vi "PDF_Interface_PDF Protokoll EPA1065_520 Pre Test.vi"(8 "error in (no error)":errorcluster caption="Fehler (Eingang, kein Fehler)", 10 "ResultPictures":T1, 11 "Save PDF File Path":path) -> (0 "error out":errorcluster caption="Fehler (Ausgang)")   [LabVIEW 2020, in "EPA 1065.lvlib" / "Pre-test verification 1065-520.lvlib"]
uses:
  Pre-test verification 1065-520.lvlib
  T90 1065-308/Ergebnis.ctl
  PDF_Interface/PDF Interface Helper/PDFResultPictures.ctl
  Sprachverwaltung/FGV Aktion Tabelle zerlegen.ctl
  Seiten/FT-IR/FGV FT-IR Aktionen.ctl
  Seiten/System Einstellungen V2/Aktioen FGV System Konstanten.ctl
  Aktion FGV Pre Test Daten.ctl
  PDF_Interface/PDF Protokoll Standard Kopf Optionen.ctl
  <vilib>/Simplicity AI/SAI_PDF_API/Classes/Context/Controls/SAI_PDF_PDF Details.ctl
  PDF_Interface/PDF Interface Helper/PDFContentType.ctl
  PDF_Interface/PDF Interface Helper/PDFTableContentType.ctl
  PDF_Interface/PDF Interface Helper/PDFResults.ctl
  PDF_Interface/PDF Interface Helper/PDFCommentPosition.ctl
  PDF_Interface/PDF Interface Helper/PDFPageBreak.ctl
  PDF_Interface/PDF Interface Helper/PDFTablePictures.ctl
  PDF_Interface/PDF Interface Helper/PDFBemerkung.ctl
  <vilib>/Simplicity AI/SAI_PDF_API/Classes/Context/Controls/SAI_PDF_Text Align.ctl
  <vilib>/Simplicity AI/SAI_PDF_API/Classes/Context/Controls/SAI_PDF_Font.ctl
  <vilib>/Simplicity AI/SAI_PDF_API/Classes/Context/Controls/SAI_PDF_Font Encoding.ctl
  Allgemein/allgemeine Sub-VIs.lvlib
  Seiten/FT-IR/FT-IR.lvlib
  Seiten/System Einstellungen V2/System Einstellungen V2.lvlib
  Sprachverwaltung/Sprachverwaltung.lvlib
  PDF_Interface/PDF Interface.lvlib
  PDF_Interface/PDF Interface Helper/PDF Interface Helper.lvlib
  <vilib>/Simplicity AI/SAI_PDF_API/Classes/Context/Context.lvclass
  Linearisierung V2/Protokoll/Protokoll.lvlib
  T90 1065-308/T90 Test 1065-308.lvlib
panel:
  out "Einheit Genauigkeit 2":string
  out "Ergebnis":T2 caption="Ergebnis 1"
  out "Ergebnis THC":string
  out "Grenze":string caption="Grenzwert:"
  out "Einheit Genauigkeit":string
  out "Versa Serial number:":string caption="Seriennummer:"
  out "Anlage:":string
  out "Methode (Recipe):":string
  out "Date & Time:":string caption="Datum & Uhrzeit:"
  out "Ergebnis:":string
  out "Flow weighted mean:":string caption="Durchflussgew. Mittelwert:"
  out "Bearbeiter:":string
  out "Serial number:":string caption="Seriennummer:"
  out "Messgerät:":string
  # "Pre Test EPA § 1065.520"
  # "Grenzen"
  # "Ergebnis"
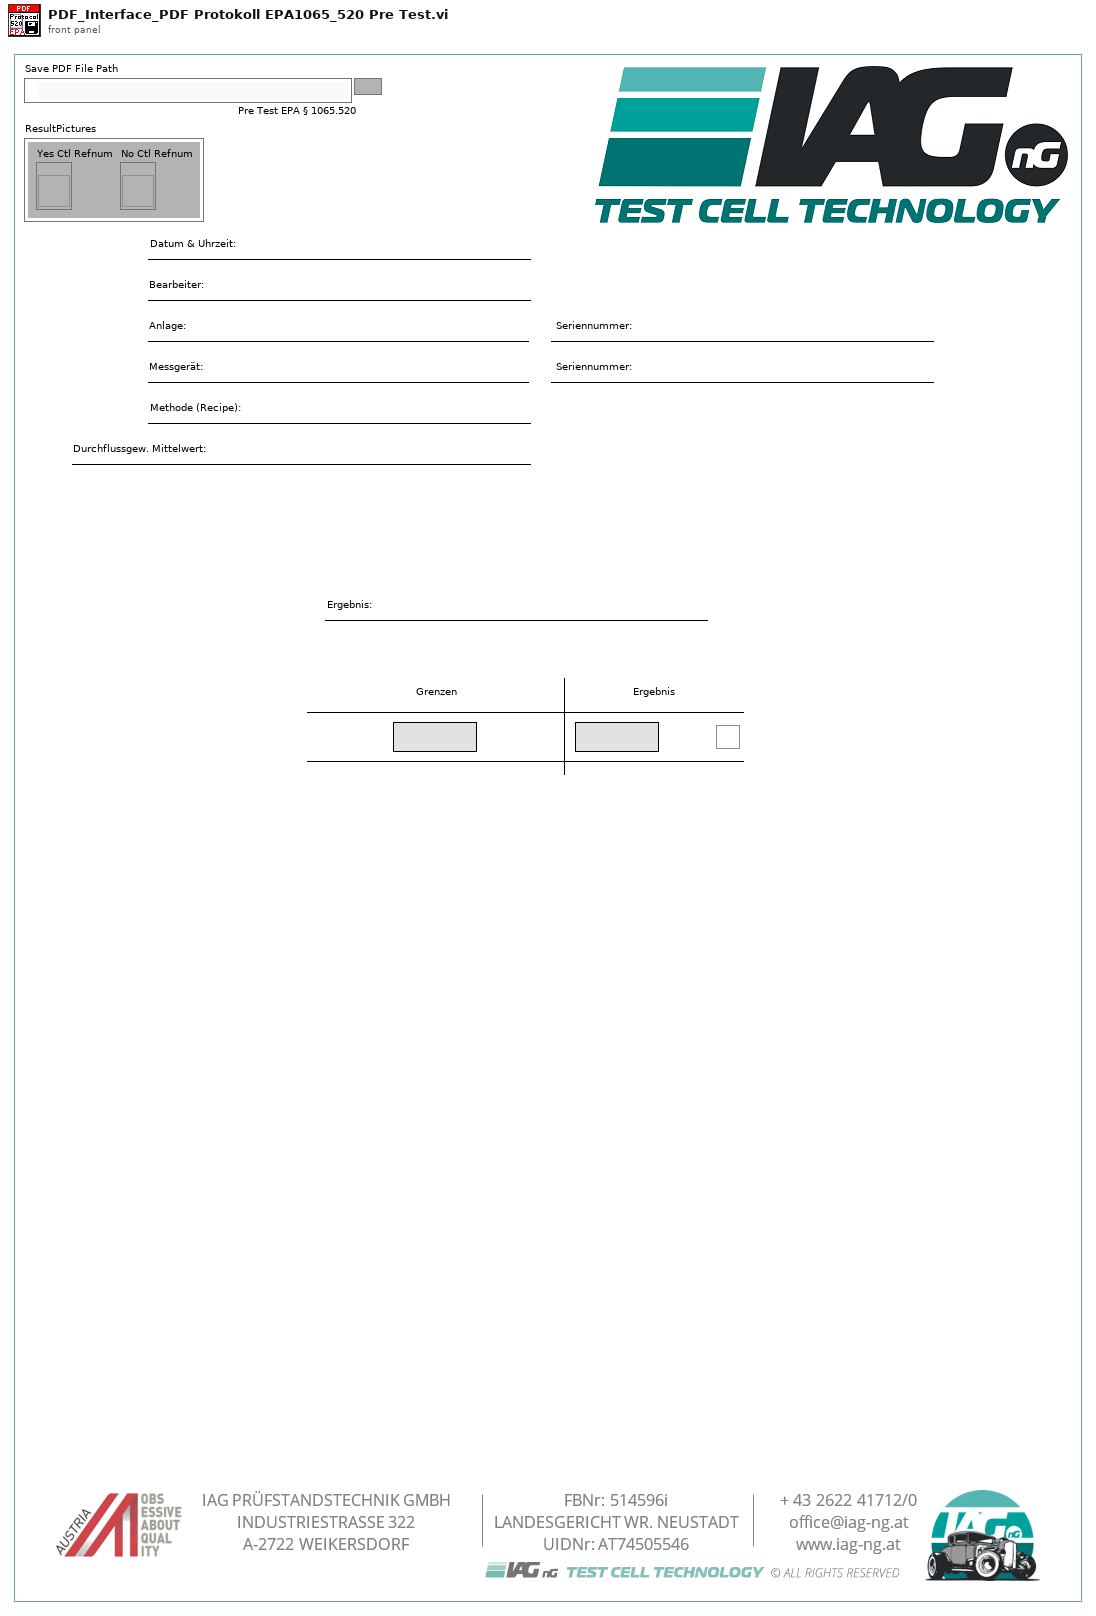
[diagram p1: front panel]
types:
  T1 = typedef "PDF Interface.lvlib/PDF Interface Helper.lvlib/PDFResultPictures.ctl" = cluster{"Yes Ctl Refnum":refnum<vi>, "No Ctl Refnum":refnum<vi>}
  T2 = typedef "EPA 1065.lvlib/T90 Test 1065-308.lvlib/Ergebnis.ctl" = bool
  T3 = typedef "Sprachverwaltung.lvlib/FGV Aktion Tabelle zerlegen.ctl" = enum16{"laden", "vereinzeln", "speichern"}
  T4 = typedef "PDF Interface.lvlib/PDF Protokoll Standard Kopf Optionen.ctl" = cluster{"Analysator":bool, "FT-IR Rezept":bool, "Gasteiler":bool, "Gas Komponente":bool, "Gas Flasche":bool, "LIN Protokoll":bool, "Operator":bool}
  T5 = typedef "EPA 1065.lvlib/Pre-test verification 1065-520.lvlib/Aktion FGV Pre Test Daten.ctl" = enum16{"lesen", "Konfig Daten", "PDF einstellen", "laden", "speichern", "Werte schreiben", "Auswerten"}
  T6 = typedef "System Einstellungen V2.lvlib/Aktioen FGV System Konstanten.ctl" = enum16{"lesen", "laden", "speichern", "Sprache"}
  T7 = typedef "FT-IR.lvlib/FGV FT-IR Aktionen.ctl" = enum16{"lesen", "NOG setzen", "NOS setzen", "Initialisieren", "speichern", "ALLES setzen", "FT-IR Spektrum loggen", "Komm Stoppen", "Spektrum LogKonfig"}
  T8 = typedef "PDF Interface.lvlib/PDF Interface Helper.lvlib/PDFResults.ctl" = cluster{"Results":cluster{"Result Text":string, "Result":bool}[], "ResultPictures":T1, "use Pictures":bool, "Image Scale (%)":sgl, "Autoscale? (T)":bool, "Horizontal Align":i32, "Position":i32}
  T9 = typedef "PDF Interface.lvlib/PDF Interface Helper.lvlib/PDFTableContentType.ctl" = cluster{"TableHeader":string[], "Table":string[][], "Relative Column Widths (%)":sgl[], "Results":T8, "PositionBemerkung":T10, "PageBreak":T11, "TablePictures":T12, "Horizontal Align":i32}
  T10 = typedef "PDF Interface.lvlib/PDF Interface Helper.lvlib/PDFCommentPosition.ctl" = enum16{"before", "after"}
  T11 = typedef "PDF Interface.lvlib/PDF Interface Helper.lvlib/PDFPageBreak.ctl" = enum16{"none", "before", "after", "after comment"}
  T12 = typedef "PDF Interface.lvlib/PDF Interface Helper.lvlib/PDFTablePictures.ctl" = cluster{"Ctl Refnum In":refnum<vi>[], "RowOrColumn":enum16{"Row", "Column"}, "IndexToInsert":u16, "Image Scale (%)":sgl[], "Autoscale? (T)":bool[], "Horizontal Align":i32}
  T13 = typedef "PDF Interface.lvlib/PDF Interface Helper.lvlib/PDFBemerkung.ctl" = cluster{"Bemerkung Text":string, "Align (Left)":T14, "Add Line Feeds (F:No)":bool, "Font":T15}
  T14 = typedef "SAI_PDF_Toolkit.lvlib/Context.lvclass/SAI_PDF_Text Align.ctl" = i32
  T15 = typedef "SAI_PDF_Toolkit.lvlib/Context.lvclass/SAI_PDF_Font.ctl" = cluster{"Font":string, "Size":i32, "Colour":u32, "Bold":bool, "Italic":bool, "Underline":bool, "Strikethrough":bool, "Font Encoding":T16}
  T16 = typedef "SAI_PDF_Toolkit.lvlib/Context.lvclass/SAI_PDF_Font Encoding.ctl" = enum16{"Cp1252, WinANSI", "IdentityH", "IdentityV", "Cp1250", "Cp1257", "MacRoman"}
  T17 = typedef "PDF Interface.lvlib/PDF Interface Helper.lvlib/PDFContentType.ctl" = cluster{"Titel":string, "Header Table":string[][], "Table Array":T9[], "Bemerkungen":T13[]}
  T18 = typedef "SAI_PDF_Toolkit.lvlib/Context.lvclass/SAI_PDF_PDF Details.ctl" = cluster{"Title":string, "Subject":string, "Keywords":string, "Author":string, "Creator":string}
  T19 = cluster{"Header Footer Text Cluster":cluster{"Header Text":string, "Footer Text":string, "Time":string, "Page Number":string}, "PDF Details":T18}
  T20 = typedef "EPA 1065.lvlib/Pre-test verification 1065-520.lvlib/Pre Konfig Daten.ctl" = cluster{"Bearbeiter:":string, "Messgerät:":string, "Seriennummer:":string, "Modus":T21, "Pfad:":path, "Textname:":string, "N2 Aufschaltzeit:":dbl, "Flow weighted mean:":dbl}
  T21 = typedef "EPA 1065.lvlib/Pre-test verification 1065-520.lvlib/Modus Pre Test.ctl" = u16
  T22 = cluster{"Modell":string, "ProjektNummer":string, "Software Version":string, "Seriennummer":string}
  T23 = cluster{"Header Size":i32, "Column Ratio left":sgl[]}
  T24 = typedef "String - Ausgabefeld.ctl" = string
  T25 = typedef "EPA 1065.lvlib/Pre-test verification 1065-520.lvlib/Pre Werte.ctl" = cluster{"THC Wert":dbl, "Berechnetes Limit":dbl, "Bestanden":bool}
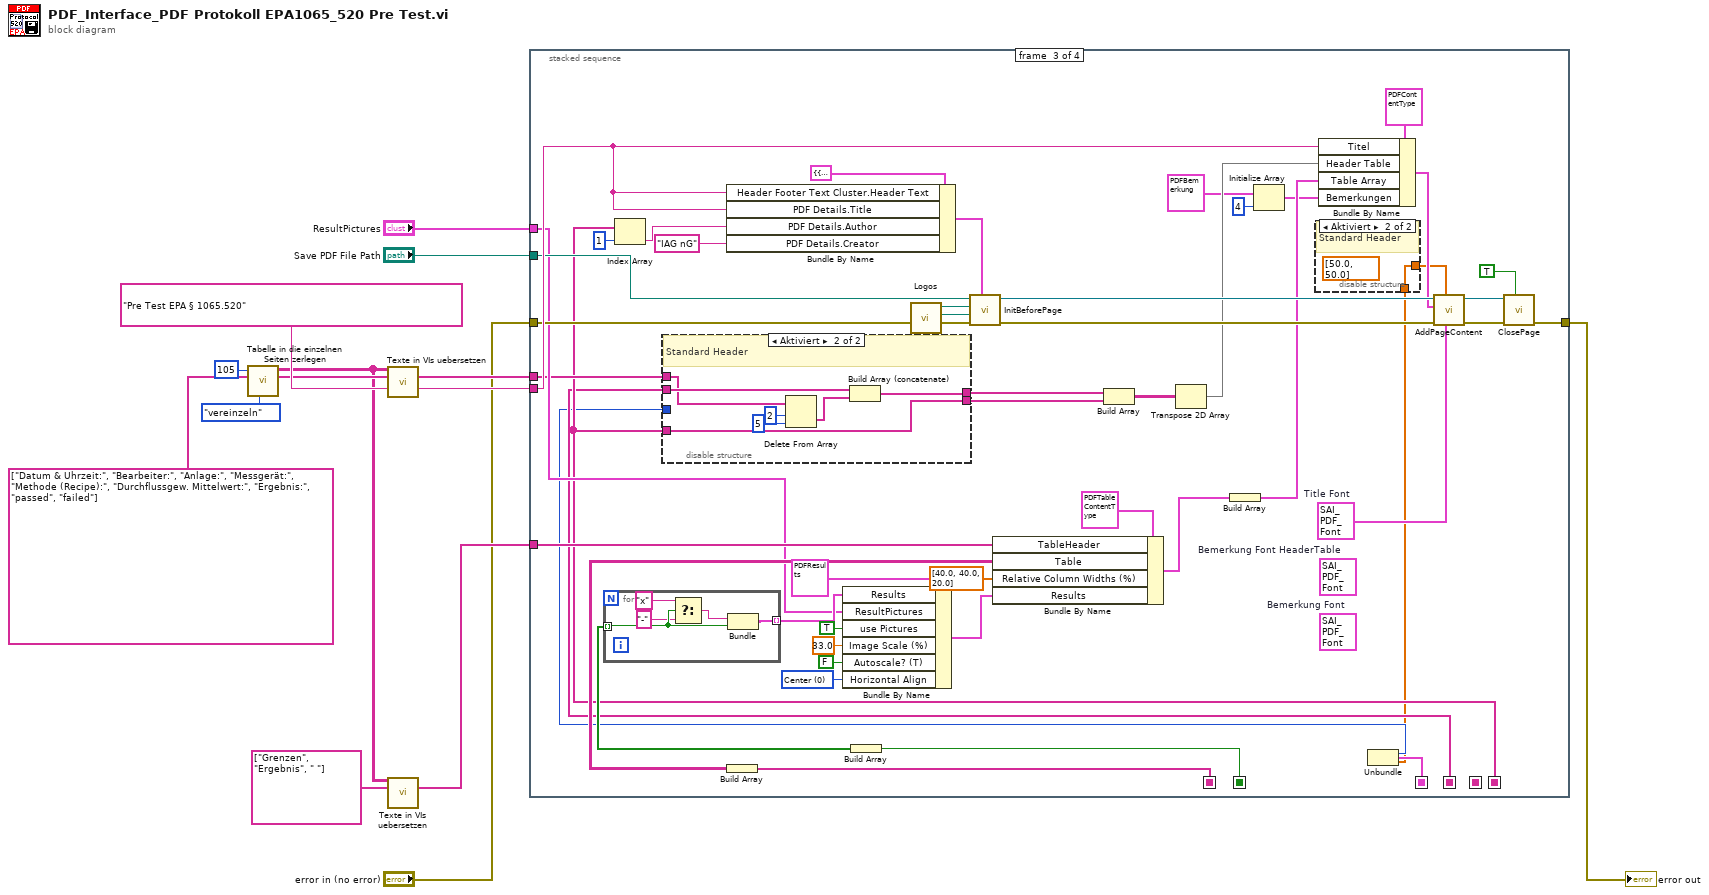
[diagram p0: block diagram]
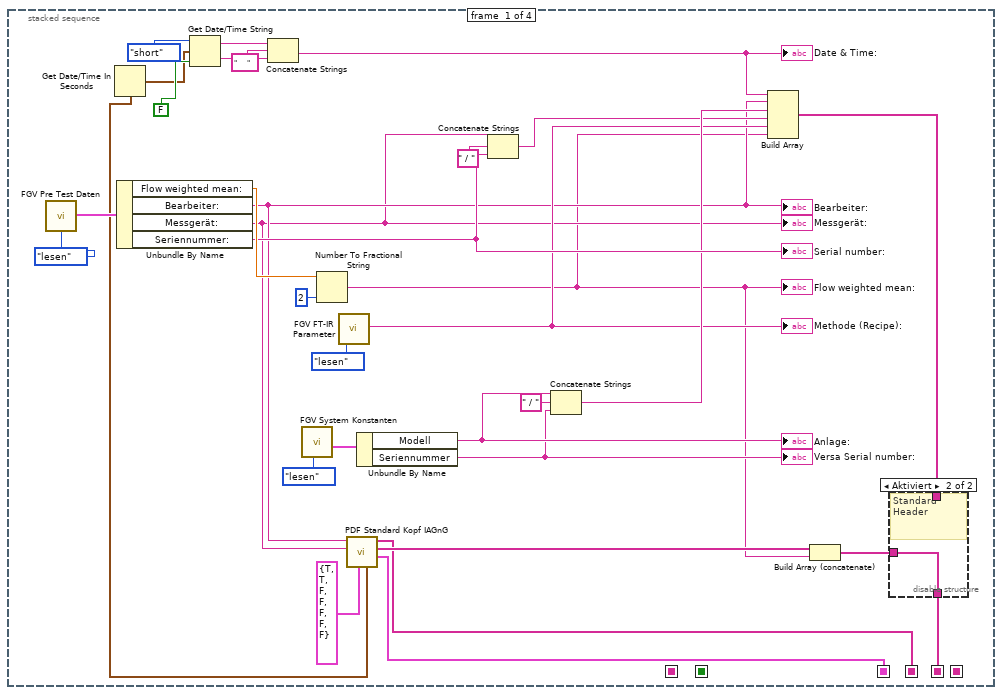
[diagram p2: hidden frame]
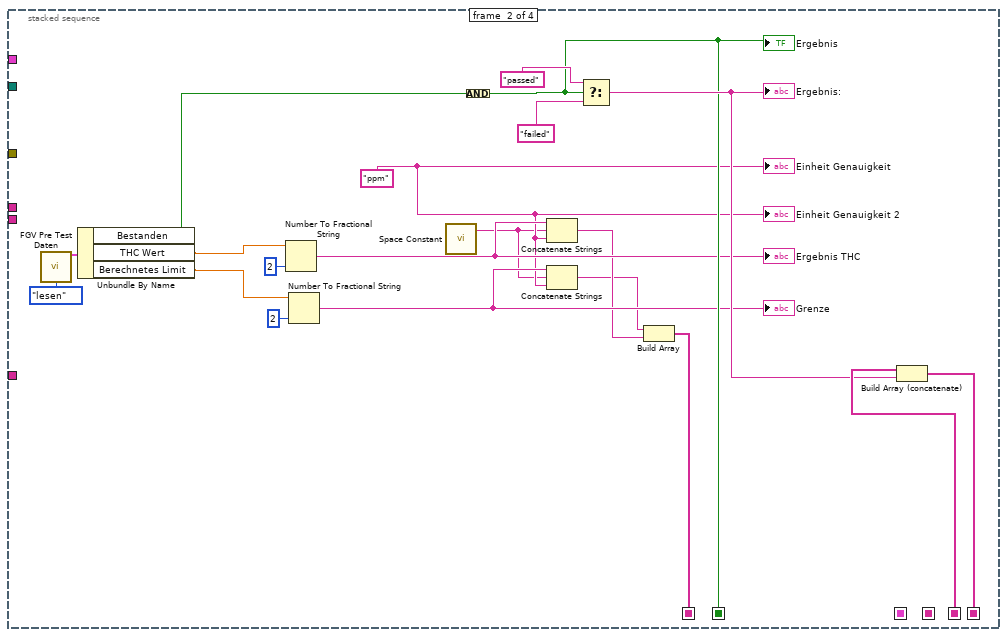
[diagram p4: hidden frame]
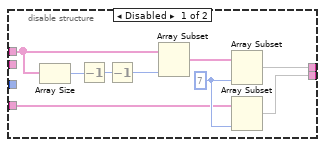
[diagram p5: hidden frame]
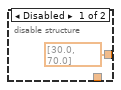
[diagram p6: hidden frame]
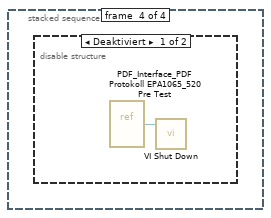
[diagram p7: hidden frame]
diagram:
  n1 = call "Tabelle in die einzelnen Seiten zerlegen.vi"("Aktion"=FGV_Aktion_Tabelle_zerlegen."vereinzeln", "Index (Seite)"=105) -> ("Sprachliste"=w5:string[][])  [unwired: 7 in, 2 out]
  n2 = call "Texte in VIs uebersetzen.vi"("Sprachliste"=w5, "String-Array zum Übersetzen"=string[] ["Datum & Uhrzeit:", "Bearbeiter:", "Anlage:", "Messgerät:", "Methode (Recipe):", "Durchflussgew. Mittelwert:", "Ergebnis:", "passed", "failed"], "String zum Übersetzen"="Pre Test EPA § 1065.520") -> ("String-Array zum Übersetzen"=w9:string[], "String zum Übersetzen"=w8:string)  [unwired: 8 in, 3 out]
  n3 = call "Texte in VIs uebersetzen.vi"("Sprachliste"=w5, "String-Array zum Übersetzen"=string[] ["Grenzen", "Ergebnis", " "]) -> ("String-Array zum Übersetzen"=w4:string[])  [unwired: 9 in, 4 out]
  n4 = stacked-sequence {
    seq-local: [w19 _ _ _] -> [_ w58 _ _]
    seq-local: [_ w56 _ _] -> [_ _ w72 _]
    seq-local: [_ w55 _ _] -> [_ _ w87 _]
    seq-local: [_ w49 _ _] -> [_ _ w86 _]
    seq-local: [w16 _ _ _] -> [_ _ w71 _]
    seq-local: [w15 _ _ _] -> [_ _ w70 _]
    tunnel: w9 -> [_ _ w73 _]
    tunnel: w8 -> [_ _ w92 _]
    tunnel: "Save PDF File Path" -> [_ _ w91 _]
    tunnel: w4 -> [_ _ w88 _]
    tunnel: "error in (no error)" -> [_ _ w90 _]
    tunnel: [_ _ w89 _] -> w2
    tunnel: "ResultPictures" -> [_ _ w78 _]
    frame #0 {
      n5 = call "FGV Pre Test Daten.vi"("Aktion"=Aktion_FGV_Pre_Test_Daten."lesen") -> ("T90 Konfig Daten 2"=w35:T20)  [unwired: 11 in, 3 out]
      n6 = Get Date/Time In Seconds() -> (seconds since 1Jan1904=w14:timestamp)
      n7 = Unbundle By Name(w35) -> ("Flow weighted mean:"=w34:dbl, "Bearbeiter:"=w23:string, "Messgerät:"=w22:string, "Seriennummer:"=w31:string)
      "Messgerät:" <- w22
      "Bearbeiter:" <- w23
      "Serial number:" <- w31
      n8 = Get Date/Time String(date format (0)=enum16{"short", "long", "abbreviated"}."short" ("Datumsformat (0)"), seconds (now)=w14, want seconds? (F)=FALSE ("Angabe von Sekunden? (F)")) -> (date string=w45:string, time string=w44:string)
      n9 = Concatenate Strings(w45, "     " ("String"), w44) -> (w33:string)
      "Date & Time:" <- w33
      n10 = call "FGV System Konstanten.vi"("Aktionen"=Aktioen_FGV_System_Konstanten."lesen") -> ("Cluster out"=w37:T22)  [unwired: 6 in, 4 out]
      n11 = Number To Fractional String(number=w34, precision (6)=i16 2 ("Genauigkeit (6)")) -> (F-format string=w20:string)  [unwired: 2 in]
      "Flow weighted mean:" <- w20
      n12 = call "FGV FT-IR Parameter.vi"("Aktion"=FGV_FT-IR_Aktionen."lesen") -> ("Current Recipe"=w25:string)  [unwired: 11 in, 7 out]
      "Methode (Recipe):" <- w25
      n13 = call "PDF Standard Kopf IAGnG.vi"("Zeitstempel"=w14, "Oprtionen Cluster"=T4 {"Analysator"=TRUE, "FT-IR Rezept"=TRUE, "Gasteiler"=FALSE, "Gas Komponente"=FALSE, "Gas Flasche"=FALSE, "LIN Protokoll"=FALSE, "Operator"=FALSE}, "Analysator"=w22, "Bearbeiter/in"=w23) -> ("Size Cluster"=w15:T23, "Header Values"=w21:T24[], "Header Labels"=w16:string[])  [unwired: 4 in, 1 out]
      n14 = Unbundle By Name(w37) -> ("Modell"=w29:string, "Seriennummer"=w28:string)
      "Versa Serial number:" <- w28
      "Anlage:" <- w29
      n15 = Concatenate Strings(w22, " / " ("String"), w31) -> (w26:string)
      n16 = Concatenate Strings(w29, " / " ("String"), w28) -> (w27:string)
      n17 = Build Array(w33, w23, w27, w26, w25, w20) -> (w18:string[])
      n18 = Build Array (concatenate)(w21, w20) -> (w17:T24[])
      n19 = disable-structure shown="Aktiviert" {
        disable-tunnel: [w46 w47] -> w19
        disable-tunnel: w18 -> [w46 _]
        disable-tunnel: w17 -> [_ w47]
        frame Disabled {
        }
        frame Enabled {
          # "Standard Header"
        }
      }
    }
    frame #1 {
      w52 = "ppm" ("Einheit Genauigkeit")
      n20 = call "FGV Pre Test Daten.vi"("Aktion"=Aktion_FGV_Pre_Test_Daten."lesen") -> ("Daten/Ergebnisse"=w62:T25)  [unwired: 11 in, 3 out]
      n21 = Unbundle By Name(w62) -> ("Bestanden"=w61:bool, "THC Wert"=w59:dbl, "Berechnetes Limit"=w60:dbl)
      n22 = Number To Fractional String(number=w59, precision (6)=i16 2 ("Genauigkeit (6)")) -> (F-format string=w54:string)  [unwired: 2 in]
      "Ergebnis THC" <- w54
      n23 = Number To Fractional String(number=w60, precision (6)=i16 2 ("Genauigkeit (6)")) -> (F-format string=w53:string)  [unwired: 2 in]
      "Grenze" <- w53
      n24 = call <vilib>:"Space Constant.vi"() -> ("String"=w48:string)
      n25 = Compound Arithmetic op=AND ("Mehrfacharithmetik")(w61) -> (w55:bool)
      "Ergebnis" <- w55
      n26 = Concatenate Strings(w54, w48, w52) -> (w51:string)
      n27 = Concatenate Strings(w53, w48, w52) -> (w50:string)
      n28 = Select(t="passed", s=w55, f="failed") -> (s? t:f=w57:string)
      "Ergebnis:" <- w57
      n29 = Build Array(w50, w51) -> (w49:string[])
      n30 = Build Array (concatenate)(w58, w57) -> (w56:T24[])
      "Einheit Genauigkeit 2" <- w52
      "Einheit Genauigkeit" <- w52
    }
    frame #2 {
      w74 = T14 0 items=["Center", "Justified", "Justified All", "Left", "Right"] ("Align (Left)")
      (unwired) T15 {"Font"="Arial", "Size"=12, "Colour"=16711680, "Bold"=TRUE, "Italic"=TRUE, "Underline"=FALSE, "Strikethrough"=FALSE, "Font Encoding"=enum."Cp1252, WinANSI"}  # Bemerkung Font HeaderTable
      (unwired) T15 {"Font"="Arial", "Size"=12, "Colour"=0, "Bold"=TRUE, "Italic"=TRUE, "Underline"=FALSE, "Strikethrough"=FALSE, "Font Encoding"=enum."Cp1252, WinANSI"}  # Bemerkung Font
      w97 = T15 {"Font"="Arial", "Size"=26, "Colour"=0, "Bold"=TRUE, "Italic"=FALSE, "Underline"=TRUE, "Strikethrough"=FALSE, "Font Encoding"=enum."Cp1252, WinANSI"}  # Title Font
      n31 = Index Array(array=w72, index=1 ("Index")) -> (element=w93:T24)
      n32 = Bundle By Name(cluster=T19 {"Header Footer Text Cluster"={"Header Text"="Protokoll XYZ", "Footer Text"="IAG nG", "Time"="<TIMESTAMP yyyy-MM-dd>", "Page Number"="Page <P> of <PT>"}, "PDF Details"={"Title"="Test PDF", "Subject"="Versa Tabasco", "Keywords"="", "Author"="RIW", "Creator"="IAG"}} ("Info"), "Header Footer Text Cluster.Header Text"=w92, "PDF Details.Title"=w92, "PDF Details.Author"=w93, "PDF Details.Creator"="IAG nG") -> (w108:T19)
      n33 = Build Array(w86) -> (w85:string[][])
      n34 = Build Array(w87) -> (w84:bool[])
      n35 = for {
        tunnel: w84 -> [w140] mode=indexing
        tunnel: [w136] -> w79 mode=indexing
        n36 = Select(t="x", s=w140, f="-") -> (s? t:f=w137:string)
        n37 = Bundle(w137, w140) -> (w136:cluster{string, bool})  [unwired: 1 in]
      }
      n38 = Bundle By Name(cluster=T8 {"Results"=[], "ResultPictures"={"Yes Ctl Refnum"=refnum, "No Ctl Refnum"=refnum}, "use Pictures"=FALSE, "Image Scale (%)"=100.0, "Autoscale? (T)"=TRUE, "Horizontal Align"=3, "Position"=0} ("Results"), "Results"=w79, "ResultPictures"=w78, "use Pictures"=TRUE, "Image Scale (%)"=sgl 33.0, "Autoscale? (T)"=FALSE, "Horizontal Align"=w74) -> (w80:T8)
      n39 = call "Logos.vi"() -> ("Footer Image File Path"=w116:path, "Header Image File Path"=w117:path)  [unwired: 8 in, 2 out]
      n40 = call "InitBeforePage.vi"("Info"=w108, "Fehler (Eingang, kein Fehler)"=w90, "Footer Image File Path"=w116, "Header Image File Path"=w117, "Path (Dialog if Empty)"=w91) -> ("Fehler (Ausgang)"=w115:errorcluster, "Context (Ausgang)"=w114:refnum<class "Context.lvclass">)  [unwired: 5 in]
      n41 = Bundle By Name(cluster=T9 {"TableHeader"=[], "Table"=[], "Relative Column Widths (%)"=[], "Results"={"Results"=[], "ResultPictures"={"Yes Ctl Refnum"=refnum, "No Ctl Refnum"=refnum}, "use Pictures"=FALSE, "Image Scale (%)"=0.0, "Autoscale? (T)"=FALSE, "Horizontal Align"=0, "Position"=0}, "PositionBemerkung"=enum."before", "PageBreak"=enum."none", "TablePictures"={"Ctl Refnum In"=[], "RowOrColumn"=enum."Row", "IndexToInsert"=0, "Image Scale (%)"=[], "Autoscale? (T)"=[], "Horizontal Align"=0}, "Horizontal Align"=0} ("Table Array"), "TableHeader"=w88, "Table"=w85, "Relative Column Widths (%)"=sgl[] [40.0, 40.0, 20.0], "Results"=w80) -> (w96:T9)
      n42 = Build Array(w96) -> (w103:T9[])
      n43 = Initialize Array(T13 {"Bemerkung Text"="", "Align (Left)"=0, "Add Line Feeds (F:No)"=FALSE, "Font"={"Font"="Arial", "Size"=10, "Colour"=0, "Bold"=FALSE, "Italic"=FALSE, "Underline"=FALSE, "Strikethrough"=FALSE, "Font Encoding"=enum."Cp1252, WinANSI"}} ("Bemerkung"), 4 ("Dimensionsgröße")) -> (w99:T13[])
      n44 = Unbundle(w70) -> ("Header Size"=w69:i32, "Column Ratio left"=w68:sgl[])
      n45 = disable-structure shown="Aktiviert" {
        disable-tunnel: [w123 w129] -> w106
        disable-tunnel: [w122 w133] -> w105
        disable-tunnel: w73 -> [w119 w131]
        disable-tunnel: w72 -> [w118 w133]
        disable-tunnel: w71 -> [_ w132]
        disable-tunnel: w69 -> [_ _]
        frame Disabled {
          w120 = 7 ("Länge")
          n46 = Array Size(array=w119) -> (size(s)=w126:i32)
          n47 = Decrement(x=w126) -> (x-1=w125:i32)
          n48 = Decrement(x=w125) -> (x-1=w124:i32)
          n49 = Array Subset(array=w119, length=w124) -> (w121:string[])  [unwired: 1 in]
          n50 = Array Subset(array=w121, length=w120) -> (w123:string[])  [unwired: 1 in]
          n51 = Array Subset(array=w118, length=w120) -> (w122:T24[])  [unwired: 1 in]
        }
        frame Enabled {
          # "Standard Header"
          n52 = Delete From Array(array=w131, length=2 ("Länge"), index=5 ("Index")) -> (deleted portion=w130:string[])  [unwired: 1 out]
          n53 = Build Array (concatenate)(w132, w130) -> (w129:string[])
        }
      }
      n54 = Build Array(w106, w105) -> (w104:T24[][])
      n55 = Transpose 2D Array(2D array=w104) -> (transposed array=w100:T24[][])
      n56 = disable-structure shown="Aktiviert" {
        disable-tunnel: [sgl[] [30.0, 70.0] ("Column Ratio left") w135] -> w101
        disable-tunnel: w68 -> [_ w135]
        frame Disabled {
        }
        frame Enabled {
          (unwired) sgl[] [50.0, 50.0] ("Column Ratio left")
          # "Standard Header"
        }
      }
      n57 = Bundle By Name(cluster=T17 {"Titel"="Test mit Graph und Results PDF", "Header Table"=[["Murks:", "4711"], ["HolyShit:", "0815"]], "Table Array"=[{"TableHeader"=["Soll\nppm/%", "Ist\nppm/%", "Fehler\n%", "Toleranz\n%", "Ergebnis"], "Table"=[["aaa", "bbb", "ccc", "ddd"], ["111", "222", "333", "444"], ["sss", "fff", "kkk", "xxx"], ["6.5", "11.13", "19.2", "4"], ["1111", "1212", "777", "888"]], "Relative Column Widths (%)"=[22.5, 22.5, 22.5, 22.5, 10.0], "Results"={"Results"=[], "ResultPictures"={"Yes Ctl Refnum"=refnum, "No Ctl Refnum"=refnum}, "use Pictures"=FALSE, "Image Scale (%)"=100.0, "Autoscale? (T)"=TRUE, "Horizontal Align"=3, "Position"=0}, "PositionBemerkung"=enum."after", "PageBreak"=enum."none", "TablePictures"={"Ctl Refnum In"=[], "RowOrColumn"=enum."Row", "IndexToInsert"=0, "Image Scale (%)"=[], "Autoscale? (T)"=[], "Horizontal Align"=3}, "Horizontal Align"=3}, {"TableHeader"=["Soll\nppm/%", "Ist\nppm/%", "Fehler\n%", "Toleranz\n%", "Ergebnis"], "Table"=[["aaa", "bbb", "ccc", "ddd"], ["111", "222", "333", "444"], ["sss", "fff", "kkk", "xxx"], ["6.5", "11.13", "19.2", "4"], ["1111", "1212", "777", "888"]], "Relative Column Widths (%)"=[22.5, 22.5, 22.5, 22.5, 10.0], "Results"={"Results"=[], "ResultPictures"={"Yes Ctl Refnum"=refnum, "No Ctl Refnum"=refnum}, "use Pictures"=FALSE, "Image Scale (%)"=100.0, "Autoscale? (T)"=TRUE, "Horizontal Align"=3, "Position"=0}, "PositionBemerkung"=enum."before", "PageBreak"=enum."before", "TablePictures"={"Ctl Refnum In"=[], "RowOrColumn"=enum."Row", "IndexToInsert"=0, "Image Scale (%)"=[], "Autoscale? (T)"=[], "Horizontal Align"=3}, "Horizontal Align"=3}, {"TableHeader"=["Soll\nppm/%", "Ist\nppm/%", "Fehler\n%", "Toleranz\n%", "Ergebnis"], "Table"=[["aaa", "bbb", "ccc", "ddd"], ["111", "222", "333", "444"], ["sss", "fff", "kkk", "xxx"], ["6.5", "11.13", "19.2", "4"], ["1111", "1212", "777", "888"]], "Relative Column Widths (%)"=[22.5, 22.5, 22.5, 22.5, 10.0], "Results"={"Results"=[], "ResultPictures"={"Yes Ctl Refnum"=refnum, "No Ctl Refnum"=refnum}, "use Pictures"=FALSE, "Image Scale (%)"=100.0, "Autoscale? (T)"=TRUE, "Horizontal Align"=3, "Position"=0}, "PositionBemerkung"=enum."before", "PageBreak"=enum."before", "TablePictures"={"Ctl Refnum In"=[], "RowOrColumn"=enum."Row", "IndexToInsert"=0, "Image Scale (%)"=[], "Autoscale? (T)"=[], "Horizontal Align"=3}, "Horizontal Align"=3}, {"TableHeader"=["Soll\nppm/%", "Ist\nppm/%", "Fehler\n%", "Toleranz\n%", "Ergebnis"], "Table"=[["aaa", "bbb", "ccc", "ddd"], ["111", "222", "333", "444"], ["sss", "fff", "kkk", "xxx"], ["6.5", "11.13", "19.2", "4"], ["1111", "1212", "777", "888"]], "Relative Column Widths (%)"=[22.5, 22.5, 22.5, 22.5, 10.0], "Results"={"Results"=[], "ResultPictures"={"Yes Ctl Refnum"=refnum, "No Ctl Refnum"=refnum}, "use Pictures"=FALSE, "Image Scale (%)"=100.0, "Autoscale? (T)"=TRUE, "Horizontal Align"=3, "Position"=0}, "PositionBemerkung"=enum."before", "PageBreak"=enum."before", "TablePictures"={"Ctl Refnum In"=[], "RowOrColumn"=enum."Row", "IndexToInsert"=0, "Image Scale (%)"=[], "Autoscale? (T)"=[], "Horizontal Align"=3}, "Horizontal Align"=3}, {"TableHeader"=["Soll\nppm/%", "Ist\nppm/%", "Fehler\n%", "Toleranz\n%", "Ergebnis"], "Table"=[["aaa", "bbb", "ccc", "ddd"], ["111", "222", "333", "444"], ["sss", "fff", "kkk", "xxx"], ["6.5", "11.13", "19.2", "4"], ["1111", "1212", "777", "888"]], "Relative Column Widths (%)"=[22.5, 22.5, 22.5, 22.5, 10.0], "Results"={"Results"=[], "ResultPictures"={"Yes Ctl Refnum"=refnum, "No Ctl Refnum"=refnum}, "use Pictures"=FALSE, "Image Scale (%)"=100.0, "Autoscale? (T)"=TRUE, "Horizontal Align"=3, "Position"=0}, "PositionBemerkung"=enum."before", "PageBreak"=enum."before", "TablePictures"={"Ctl Refnum In"=[], "RowOrColumn"=enum."Row", "IndexToInsert"=0, "Image Scale (%)"=[], "Autoscale? (T)"=[], "Horizontal Align"=3}, "Horizontal Align"=3}], "Bemerkungen"=[{"Bemerkung Text"="super geiles PDF", "Align (Left)"=0, "Add Line Feeds (F:No)"=TRUE, "Font"={"Font"="Arial", "Size"=10, "Colour"=0, "Bold"=FALSE, "Italic"=FALSE, "Underline"=FALSE, "Strikethrough"=FALSE, "Font Encoding"=enum."Cp1252, WinANSI"}}, {"Bemerkung Text"="", "Align (Left)"=0, "Add Line Feeds (F:No)"=FALSE, "Font"={"Font"="Arial", "Size"=10, "Colour"=0, "Bold"=FALSE, "Italic"=FALSE, "Underline"=FALSE, "Strikethrough"=FALSE, "Font Encoding"=enum."Cp1252, WinANSI"}}, {"Bemerkung Text"="Tabelle mit optionalen Ergebnissen", "Align (Left)"=3, "Add Line Feeds (F:No)"=FALSE, "Font"={"Font"="Arial", "Size"=10, "Colour"=0, "Bold"=FALSE, "Italic"=FALSE, "Underline"=FALSE, "Strikethrough"=FALSE, "Font Encoding"=enum."Cp1252, WinANSI"}}, {"Bemerkung Text"="Graph geht ab ... ", "Align (Left)"=0, "Add Line Feeds (F:No)"=FALSE, "Font"={"Font"="Arial", "Size"=10, "Colour"=0, "Bold"=FALSE, "Italic"=FALSE, "Underline"=FALSE, "Strikethrough"=FALSE, "Font Encoding"=enum."Cp1252, WinANSI"}}]} ("Content"), "Titel"=w92, "Header Table"=w100, "Table Array"=w103, "Bemerkungen"=w99) -> (w102:T17)
      n58 = call "AddPageContent.vi"("Title Font"=w97, "Column Ratio left"=w101, "error in"=w115, "Content"=w102, "Context (Eingang)"=w114) -> ("error out"=w113:errorcluster, "Context (Ausgang)"=w112:refnum<class "Context.lvclass">)  [unwired: 5 in]
      n59 = call "ClosePage.vi"("popup viewer"=TRUE, "Fehler (Eingang, kein Fehler)"=w113, "Context (Eingang)"=w112) -> ("Fehler (Ausgang)"=w89:errorcluster)  [unwired: 8 in]
    }
    frame #3 {
      n60 = disable-structure shown="Deaktiviert" {
        frame Disabled {
          n61 = vi-ref "PDF_Interface_PDF Protokoll EPA1065_520 Pre Test.vi"() -> (w141:refnum<vi>)
          n62 = call "VI Shut Down.vi"("VI Referenz"=w141) -> ()  [unwired: 11 in]
        }
        frame Enabled {
        }
      }
    }
  }
  "error out" <- w2
